vi "Main.vi"() -> ()   [LabVIEW 2026]
uses:
  <vilib>/xnet/xnet.llb/XNET Example IP Stack Config - Simple VLAN.ctl
panel:
  in  "Log Results":bool
  in  "Listen Port":u16=6341
  in  "Direction":string(combo)="outbound"
  in  "Protocol":string(combo)="tcp"
  in  "Sleep Capability":enum16{"Disabled", "Enabled"}(ring)
  in  "Speed":enum16{"1000Mb/s", "100Mb/s"}(ring)
  in  "Port Configuration":T1[](array[typedef])
  in  "DUT Password":string="nitest"
  in  "DUT Username":string="Administrator"
  in  "Client_adapter_IP_remote":string="192.168.1.3" caption="DUT IP"
  out "Ping":bool
  in  "XNET Interface":refnum<k21>="ENET1"
  out "Server results":T2
  out "Client results":T2
  in  "iPerf Test":bool
  out "Link Status":T3
  in  "Ping Test":bool
  in  "PuTTY root folder":path=path "C:/DEV/emea-tra-iPerf_bus_load_test/utility/Putty_ssh_client"
  in  "iPerf_path_remote_client":path=path "C:/DEV/emea-tra-iPerf_bus_load_test/utility/iperf3.17.1_64" caption="iPerf root folder CLIENT"
  in  "iPerf_path_remote_server":path=path "C:/DEV/emea-tra-iPerf_bus_load_test/utility/iperf3.17.1_64" caption="iPerf root folder SERVER"
  in  "Stack mode":enum16{"OS stack", "IP stack"}(ring)
  in  "Port client":i32=61000 min=1
  in  "Port server":i32=62000 min=1
  in  "Protocol":enum16{"UDP", "TCP"}(ring)=enum."TCP"
  in  "Force traffic (UDP only)":T4(ring)
  in  "iPerf sending duration":i32=10 min=1 format="%.0f sec"
  # "Interface Parameters"
  # "DUT Parameters"
  # "Status"
  # "iPerf"
  # "NOTES:\nContinuous or time bound."
  # "Target Port ssh\nTarget Port"
  # "iPerf Test Settings"
  # "Proxy Configuration"
  # "Tests"
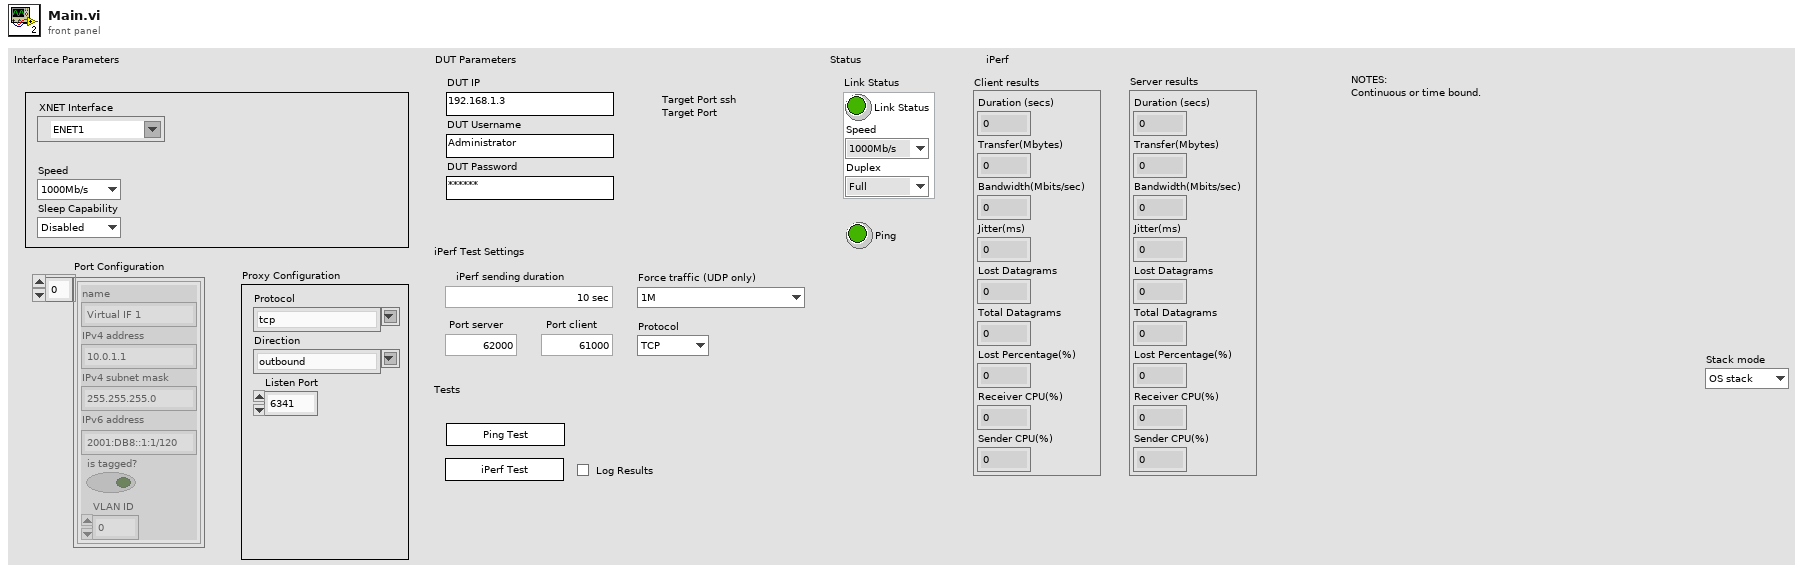
[diagram p1: front panel]
types:
  T1 = typedef "XNET Example IP Stack Config - Simple VLAN.ctl" = cluster{"name":string, "IPv4 address":string, "IPv4 subnet mask":string, "IPv6 address":string, "is tagged?":bool, "VLAN ID":u16}
  T2 = cluster{"Duration (secs)":dbl, "Transfer(Mbytes)":dbl, "Bandwidth(Mbits/sec)":dbl, "Jitter(ms)":dbl, "Lost Datagrams":i32, "Total Datagrams":i32, "Lost Percentage(%)":dbl, "Receiver CPU(%)":dbl, "Sender CPU(%)":dbl}
  T3 = cluster{"Link Status":bool, "Speed":enum16{"1000Mb/s", "100Mb/s"}, "Duplex":enum16{"Full", "Half"}}
  T4 = enum16{"1M", "10M", "20M", "30M", "40M", "50M", "100M", "500M", "1000M"}
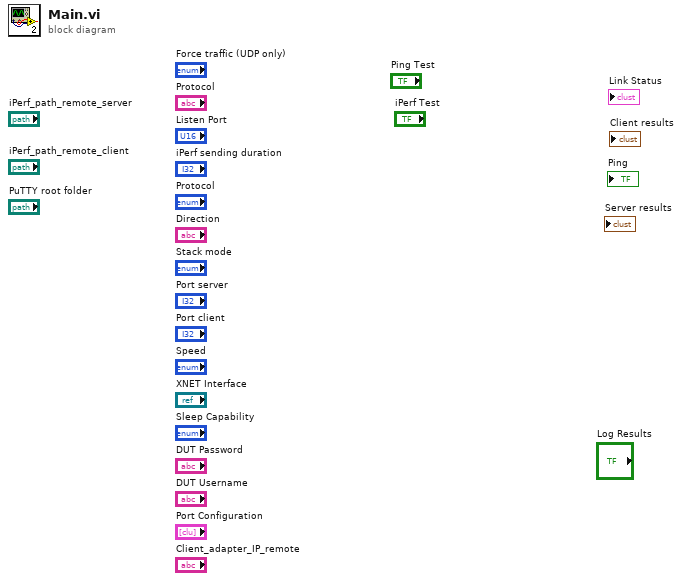
[diagram p0: block diagram]
diagram:
